vi "grain_coords_from_ROI.vi"(8 "Error In":errorcluster, 11 "ROI In":T1) -> (0 "Error Out":errorcluster, 2 "y":dbl, 3 "x":dbl)   [LabVIEW 2019]
doc: "Calcualte the grain center coordinates from the ROI global rectangle."
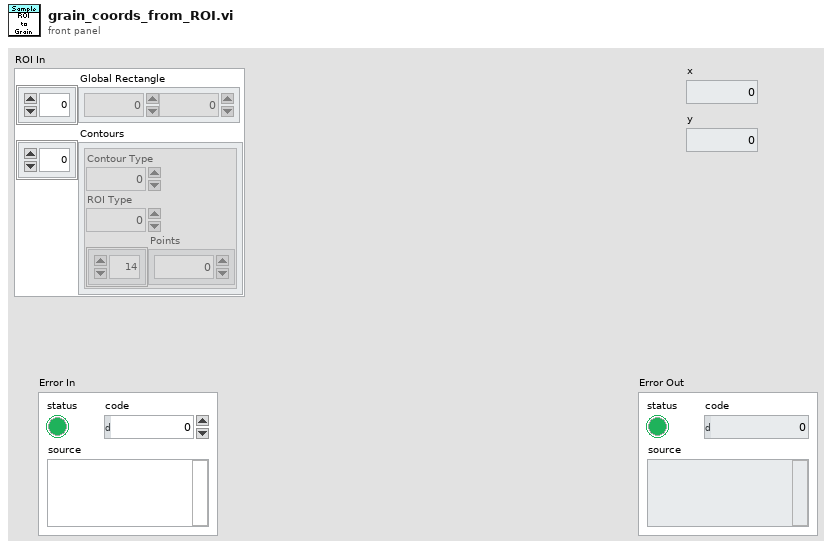
[diagram p1: front panel]
types:
  T1 = cluster{"Global Rectangle":i32[], "Contours":cluster{"Contour Type":u32, "ROI Type":u32, "Points":i32[]}[]}
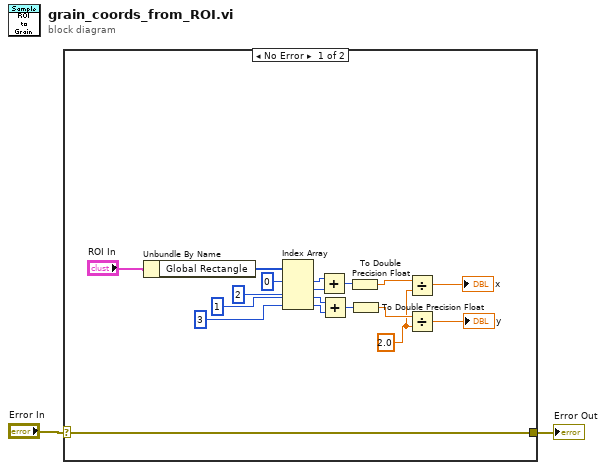
[diagram p0: block diagram]
diagram:
  n1 = case shown="No Error" "Error In" {
    selector: "Error In" -> [w20 w21]
    tunnel: [w20 w21] -> w1
    frame No Error {
      w5 = 2.0 ("y")
      n2 = Unbundle By Name("ROI In") -> ("Global Rectangle"=w18:i32[])
      n3 = Index Array(array=w18, index #1=0 ("index"), index #2=2 ("index"), index #3=1 ("index"), index #4=3 ("index")) -> (element #1=w12:i32, element #2=w13:i32, element #3=w11:i32, element #4=w10:i32)
      n4 = Add(x=w12, y=w13) -> (x+y=w9:i32)
      n5 = Add(x=w11, y=w10) -> (x+y=w8:i32)
      n6 = To Double Precision Float(number=w9) -> (double precision float=w7:dbl)
      n7 = To Double Precision Float(number=w8) -> (double precision float=w6:dbl)
      n8 = Divide(x=w7, y=w5) -> (x/y=→"x":dbl)
      n9 = Divide(x=w6, y=w5) -> (x/y=→"y":dbl)
    }
    frame Error {
    }
  }
  "Error Out" <- w1
